vi "Init.vi"(8 "error in (no error)":errorcluster, 9 "Div bit rate":dbl=32.0, 10 "Carrier":dbl=13560.0, 11 "ISO 14443 A DOWN in":refnum<class "ISO 14443 A DOWN.lvclass">) -> (0 "error out":errorcluster, 3 "ISO 14443 A DOWN out":refnum<class "ISO 14443 A DOWN.lvclass">)   [LabVIEW 2019]
uses:
  ISO 14443 A DOWN.lvclass
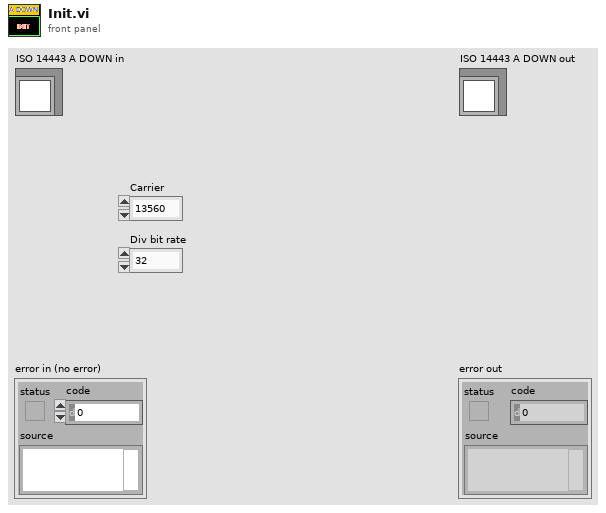
[diagram p1: front panel]
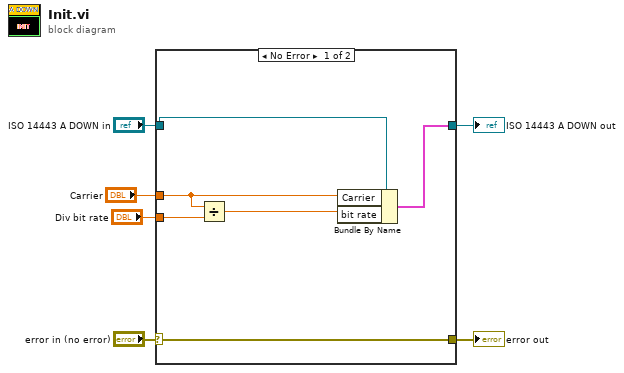
[diagram p0: block diagram]
diagram:
  n1 = case shown="No Error" "error in (no error)" {
    selector: "error in (no error)" -> [w12 w14]
    tunnel: [w12 w14] -> w5
    tunnel: "ISO 14443 A DOWN in" -> [w11 w13]
    tunnel: [w10 w13] -> w3
    tunnel: "Carrier" -> [w9 _]
    tunnel: "Div bit rate" -> [w8 _]
    frame No Error {
      n2 = Divide(x=w9, y=w8) -> (x/y=w7:dbl)
      n3 = Bundle By Name(cluster=w11, "Carrier"=w9, "bit rate"=w7) -> (w10:cluster{})
    }
    frame Error {
    }
  }
  "error out" <- w5
  "ISO 14443 A DOWN out" <- w3
